vi "Colour sorting machine(all modules combined).vi"() -> ()   [LabVIEW 2018]
uses:
  <vilib>/userdefined/High Color/IMAQdx.ctl
  <vilib>/myRIO/Instrument Drivers/Onboard IO/DIO/typedefs/DIO Reference.ctl
  <vilib>/myRIO/Common/Instrument Driver Framework/Utilities/typedefs/myRIO Generic Hardware Reference.ctl
  <vilib>/myRIO/Common/Instrument Driver Framework/Utilities/typedefs/Hardware Version Enum.ctl
  <vilib>/myRIO/Common/Instrument Driver Framework/Utilities/typedefs/myRIO v1.0 Reference.ctl
  <vilib>/myRIO/Common/Instrument Driver Framework/Utilities/typedefs/Generic FPGA Reference.ctl
  <vilib>/myRIO/Common/Instrument Driver Framework/myRIO v1.0/DIO/typedefs/DIO Channels List.ctl
  <vilib>/myRIO/Common/Instrument Driver Framework/myRIO v1.0/DIO/typedefs/DIO Channels Enum.ctl
  <vilib>/userdefined/High Color/nirio_resource_hc.ctl
  <vilib>/myRIO/Instrument Drivers/Onboard IO/PWM/typedefs/PWM Reference.ctl
  <vilib>/myRIO/Common/Instrument Driver Framework/myRIO v1.0/PWM/typedefs/PWM Channels Enum.ctl
  <vilib>/myRIO/Instrument Drivers/Onboard IO/PWM/typedefs/PWM Configuration.ctl
  <vilib>/myRIO/Common/Instrument Driver Framework/Utilities/vis/Is FPGA Ref Available.vi
  <vilib>/myRIO/Common/Instrument Driver Framework/myRIO v1.0/DIO/vis/myRIO v1.1 Open DIO.vi
  <vilib>/myRIO/Instrument Drivers/Onboard IO/DIO/vis/Write.vi
  <vilib>/myRIO/Common/Instrument Driver Framework/myRIO v1.0/PWM/vis/myRIO v1.1 Open PWM.vi
  <vilib>/myRIO/Instrument Drivers/Onboard IO/PWM/vis/Set Duty Cycle and Frequency.vi
  <vilib>/myRIO/Common/Instrument Driver Framework/Utilities/vis/Validate Channels.vi
  <vilib>/myRIO/Common/Instrument Driver Framework/myRIO v1.0/DIO/vis/myRIO v1.0 Reserve DIO.vi
  <vilib>/myRIO/Common/Instrument Driver Framework/myRIO v1.0/PWM/vis/myRIO v1.0 Reserve PWM.vi
  <vilib>/myRIO/Common/Instrument Driver Framework/myRIO v1.0/Resource Manager/vis/myRIO v1.0 Reserve Channel List.vi
  <vilib>/myRIO/Common/Instrument Driver Framework/myRIO v1.0/DIO/vis/myRIO v1.0 Build MUX Configuration DIO.vi
  <vilib>/myRIO/Common/Instrument Driver Framework/myRIO v1.0/PWM/vis/myRIO v1.0 Build MUX Configuration PWM.vi
  <vilib>/myRIO/Common/Instrument Driver Framework/myRIO v1.0/Resource Manager/vis/myRIO v1.0 Reserve Channel.vi
  <vilib>/myRIO/Common/Instrument Driver Framework/myRIO v1.0/Resource Manager/vis/myRIO v1.0 Unreserve Channel.vi
  <vilib>/myRIO/Common/Instrument Driver Framework/myRIO v1.0/Resource Manager/vis/myRIO v1.0 Create Configuration List.vi
  <vilib>/myRIO/Common/Instrument Driver Framework/myRIO v1.0/Resource Manager/vis/myRIO v1.0 Build Mutex Name.vi
  <vilib>/Utility/VariantDataType/GetNumericInfo.vi
  <vilib>/Utility/error.llb/Error Cluster From Error Code.vi
  <vilib>/myRIO/Common/Instrument Driver Framework/myRIO v1.0/myRIO v1.1 Open.vi
  <vilib>/myRIO/Common/Instrument Driver Framework/Utilities/vis/IO Manager.vi
  <vilib>/myRIO/Common/Instrument Driver Framework/Utilities/vis/Configuration Manager.vi
  <vilib>/myRIO/Common/Instrument Driver Framework/myRIO v1.0/Resource Manager/vis/myRIO v1.0 Configure IO.vi
  <vilib>/myRIO/Common/Instrument Driver Framework/myRIO v1.0/myRIO v1.0 Close.vi
  <vilib>/myRIO/Common/Instrument Driver Framework/myRIO v1.0/DIO/vis/myRIO v1.0 Write DIO.vi
  <vilib>/myRIO/Common/Instrument Driver Framework/myRIO v1.0/PWM/vis/myRIO v1.0 Write PWM.vi
  <vilib>/myRIO/Express VI/Onboard IO/DO/DO Express VI.xnode
  <vilib>/myRIO/Instrument Drivers/Onboard IO/DIO/vis/myRIO DIO Open.xnode
  <vilib>/myRIO/Express VI/Onboard IO/PWM/PWM Express VI.xnode
  <vilib>/myRIO/Instrument Drivers/Onboard IO/PWM/vis/myRIO PWM Open.xnode
  <vilib>/myRIO/Instrument Drivers/Onboard IO/DIO/DIO.lvlib
  <vilib>/myRIO/Instrument Drivers/Onboard IO/PWM/PWM.lvlib
  <vilib>/vision/driver/NI_Vision_Acquisition_Software.lvlib
  <vilib>/vision/NI_Vision_Development_Module.lvlib
panel:
  out "Image":T1(plugin-control)
  out "red":bool
  out "blue":bool
  out "green":bool
  in  "Color Sensitivity":u32(ring) items=["Low", "Medium", "High"]
  out "Color Spectrum":dbl[](array[numeric]) format="%.2f"
  in  "Frequency [Hz]":dbl=1000.0
  in  "Duty Cycle":dbl=0.5297619047619048
  out "Numeric 3":i32
  out "x = y?":bool
  out "Numeric 2":i32
  out "Boolean":bool
  in  "stop":bool
  # "green"
  # "red"
  # "blue"
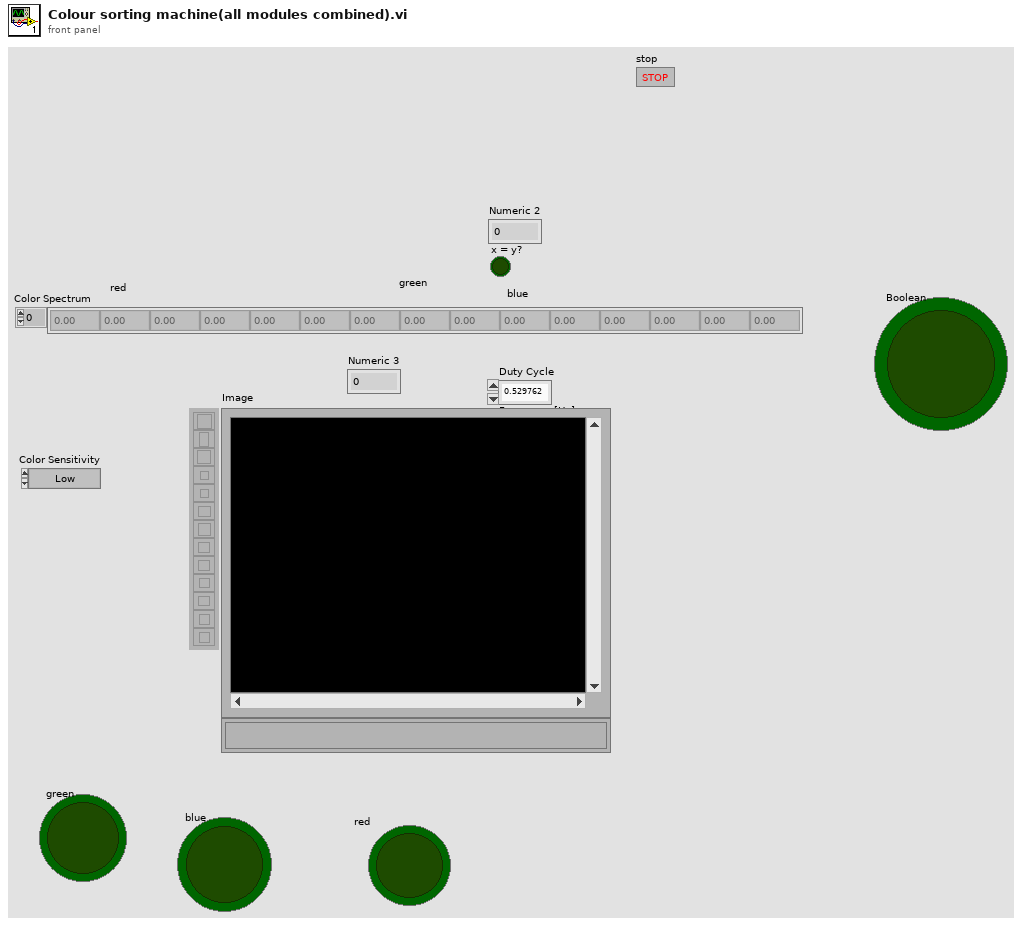
[diagram p1: front panel]
types:
  T1 = typedef "IMAQ Image.ctl" = refnum<image>
  T2 = typedef "IMAQdx.ctl" = refnum<k21>
  T3 = typedef "DIO.lvlib/DIO Reference.ctl" = cluster{"myRIO Reference":T4, "DIO Channels List":T8}
  T4 = typedef "myRIO Generic Hardware Reference.ctl" = cluster{"myRIO Model":T5, "myRIO Hardware Reference":T6}
  T5 = typedef "Hardware Version Enum.ctl" = enum16{"Unknown", "myRIO-1900", "myRIO-1950", "roboRIO", "NI ELVIS RIO CM", "ELVIS III"}
  T6 = typedef "myRIO v1.0 Reference.ctl" = cluster{"Generic FPGA Reference":T7, "Allow multiple opens":bool}
  T7 = typedef "Generic FPGA Reference.ctl" = refnum<k20>
  T8 = typedef "DIO Channels List.ctl" = T9[]
  T9 = typedef "DIO Channels Enum.ctl" = enum16{"Not Connected", "C/DIO0", "C/DIO1", "C/DIO2", "C/DIO3", "C/DIO4", "C/DIO5", "C/DIO6", "C/DIO7", "A/DIO0", "A/DIO1", "A/DIO2", "A/DIO3", "A/DIO4", "A/DIO5", "A/DIO6", "A/DIO7", "A/DIO8", "A/DIO9", "A/DIO10", "A/DIO11", "A/DIO12", "A/DIO13", "A/DIO14", "A/DIO15", "A/DIO16", "A/DIO17", "A/DIO18", "A/DIO19", "B/DIO0", "B/DIO1", "B/DIO2", "B/DIO3", "B/DIO4", "B/DIO5", "B/DIO6", "B/DIO7", "B/DIO8", "B/DIO9", "B/DIO10", "B/DIO11", "B/DIO12", "B/DIO13", "B/DIO14", "B/DIO15", "B/DIO16", "B/DIO17", "B/DIO18", "B/DIO19", "LED0", "LED1", "LED2", "LED3", "Button0", "DIO/DIO0", "DIO/DIO1", "DIO/DIO2", "DIO/DIO3", "DIO/DIO4", "DIO/DIO5", "DIO/DIO6", "DIO/DIO7", "DIO/DIO8", "DIO/DIO9", "SPI/CS0", "SPI/CS1", "SPI/CS2", "SPI/CS3", "LED RADIO (Green)", "LED RADIO (Red)", "LED COMM (Green)", "LED COMM (Red)", "LED MODE (Green)", "LED MODE (Red)"}
  T10 = typedef "nirio_resource_hc.ctl" = tag
  T11 = typedef "PWM.lvlib/PWM Reference.ctl" = cluster{"myRIO Reference":T4, "PWM Channels Enum":T12, "PWM Configuration":T13}
  T12 = typedef "PWM Channels Enum.ctl" = enum16{"Not Connected", "C/PWM0", "C/PWM1", "A/PWM0", "A/PWM1", "A/PWM2", "A/PWM3", "A/PWM4", "A/PWM5", "A/PWM6", "A/PWM7", "A/PWM8", "A/PWM9", "A/PWM10", "A/PWM11", "A/PWM12", "A/PWM13", "A/PWM14", "A/PWM15", "A/PWM16", "A/PWM17", "A/PWM18", "A/PWM19", "B/PWM0", "B/PWM1", "B/PWM2", "B/PWM3", "B/PWM4", "B/PWM5", "B/PWM6", "B/PWM7", "B/PWM8", "B/PWM9", "B/PWM10", "B/PWM11", "B/PWM12", "B/PWM13", "B/PWM14", "B/PWM15", "B/PWM16", "B/PWM17", "B/PWM18", "B/PWM19", "PWM/PWM0", "PWM/PWM1", "PWM/PWM2", "PWM/PWM3", "PWM/PWM4", "PWM/PWM5", "PWM/PWM6", "PWM/PWM7", "PWM/PWM8", "PWM/PWM9"}
  T13 = typedef "PWM.lvlib/PWM Configuration.ctl" = cluster{"Frequency":dbl, "Duty Cycle":dbl}
  T14 = cluster{"Global Rectangle":i32[], "Contours":cluster{"Contour Type":u32, "ROI Type":u32, "Points":i32[]}[]}
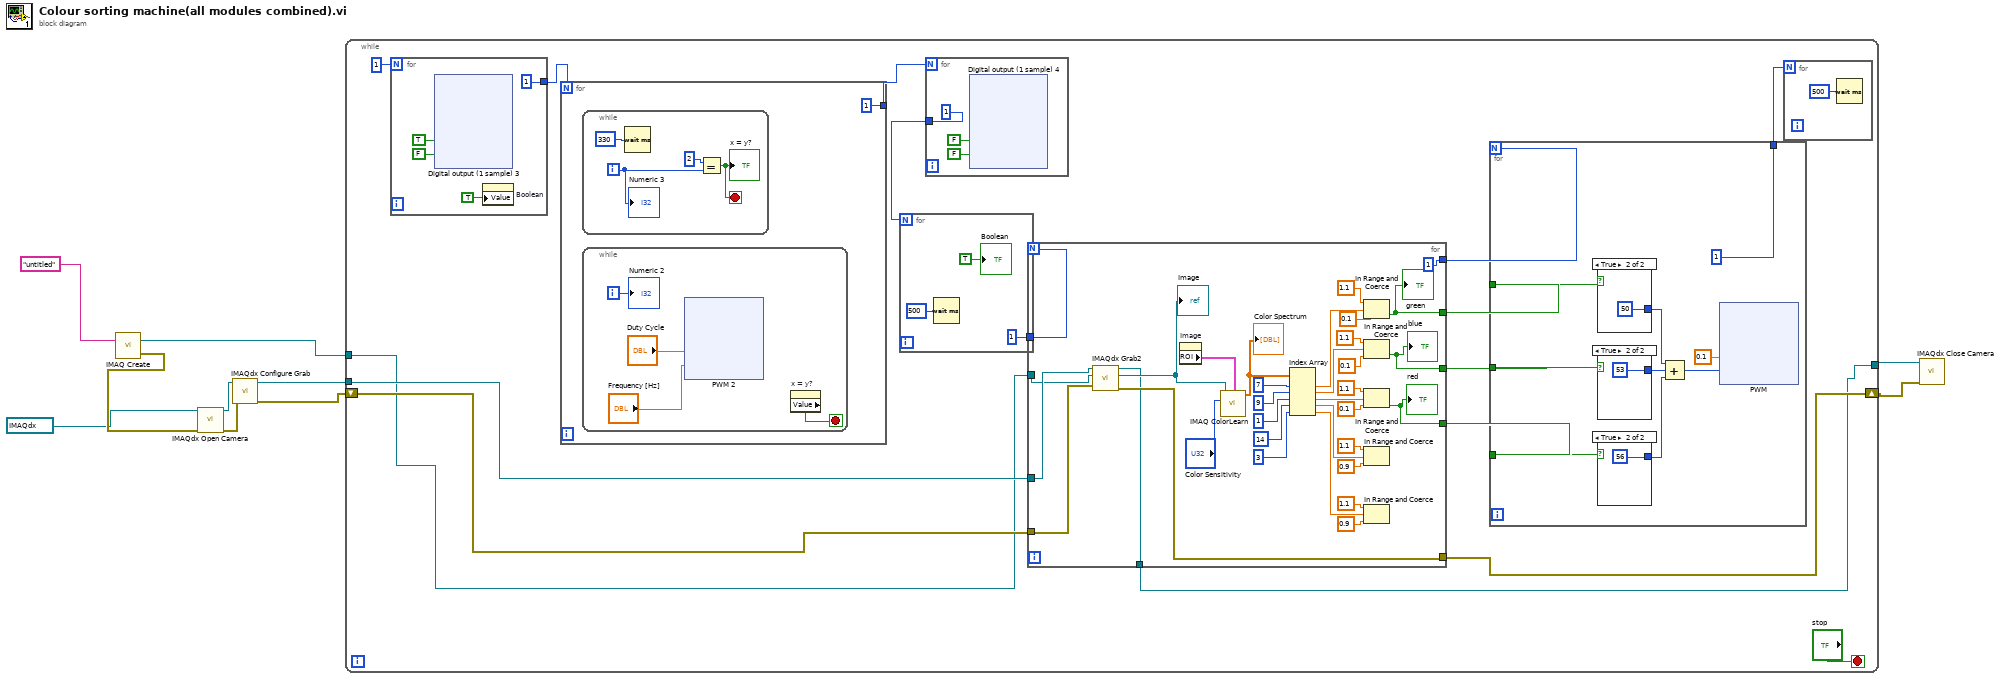
[diagram p0: block diagram]
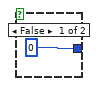
[diagram p4: hidden frame]
diagram:
  n1 = call "IMAQ Create"("Image Name"="untitled") -> ("New Image"=w3:T1, "error out"=w10:errorcluster)  [unwired: 4 in]
  n2 = call <vilib>:"IMAQdx Open Camera.vi"("error in"=w10, "Session In"=T2 "cam0") -> ("error out"=w8:errorcluster, "Session Out"=w9:T2)  [unwired: 8 in]
  n3 = call <vilib>:"IMAQdx Configure Grab.vi"("error in"=w8, "Session In"=w9) -> ("error out"=w5:errorcluster, "Session Out"=w4:T2)  [unwired: 8 in]
  n4 = while {
    shift-right: [w17] -> w2
    shift-left: w5 -> [w20]
    tunnel: w4 -> [w19]
    tunnel: w3 -> [w18]
    tunnel: [w16] -> w1
    stop <- "stop" stop-if-true
    n5 = for {
      N: 1 -> [_]
      tunnel: [1] -> w23
      n6 = xnode "Digital output (1 sample) 3"("clock (B/DIO0 (Pin 11))"=TRUE, "AntiClock (B/DIO1 (Pin 13))"=FALSE) -> ()  [unwired: 1 in, 1 out]
      n7 = property on="Boolean" class="Bool (strict)"("Value"=TRUE) -> ()  [unwired: 2 in, 2 out]
    }
    n8 = for {
      N: w23 -> [_]
      tunnel: [1] -> w22
      n9 = while {
        i -> [w70]
        stop <- w68 stop-if-true
        n10 = Wait (ms)(milliseconds to wait=u32 330) -> ()  [unwired: 1 out]
        n11 = Equal?(x=2, y=w70) -> (x = y?=w68:bool)
        "x = y?" <- w68
        "Numeric 3" <- w70
      }
      n12 = while {
        i -> [w75]
        stop <- w74 stop-if-true
        n13 = xnode "PWM 2"("Duty Cycle"="Duty Cycle", "Frequency [Hz]"="Frequency [Hz]") -> ()  [unwired: 1 in, 1 out]
        n14 = property on="x = y?" class="Bool (strict)"() -> ("Value"=w74:bool)  [unwired: 2 in, 2 out]
        "Numeric 2" <- w75
      }
    }
    n15 = for {
      N: w22 -> [_]
      tunnel: [1] -> w15
      n16 = xnode "Digital output (1 sample) 4"("clock (B/DIO0 (Pin 11))"=FALSE, "AntiClock (B/DIO1 (Pin 13))"=FALSE) -> ()  [unwired: 1 in, 1 out]
    }
    n17 = for {
      N: w15 -> [_]
      tunnel: [1] -> w25
      n18 = Wait (ms)(milliseconds to wait=u32 500) -> ()  [unwired: 1 out]
      "Boolean" <- TRUE
    }
    n19 = for {
      N: w25 -> [_]
      tunnel: [1] -> w21
      tunnel: w20 -> [w211]
      tunnel: w19 -> [w210]
      tunnel: w18 -> [w209]
      tunnel: [w208] -> w17
      tunnel: [w207] -> w16
      tunnel: [w206] -> w14
      tunnel: [w205] -> w13
      tunnel: [w204] -> w12
      n20 = call <vilib>:"IMAQdx Grab2.vi"("error in"=w211, "Image In"=w209, "Session In"=w210) -> ("error out"=w208:errorcluster, "Image Out"=w214:T1, "Session Out"=w207:T2)  [unwired: 5 in, 1 out]
      "Image" <- w214
      n21 = property on="Image" class="ImageControl"() -> ("ROI"=w213:T14)  [unwired: 2 in, 2 out]
      n22 = call "IMAQ ColorLearn"("ROI Descriptor"=w213, "Image"=w214, "Color Sensitivity"="Color Sensitivity") -> ("Color Spectrum"=w233:dbl[])  [unwired: 5 in, 1 out]
      "Color Spectrum" <- w233
      n23 = Index Array(array=w233, index #1=7 ("index"), index #2=9 ("index"), index #3=1 ("index"), index #4=14 ("index"), index #5=3 ("index")) -> (element #1=w203:dbl, element #2=w226:dbl, element #3=w223:dbl, element #4=w220:dbl, element #5=w218:dbl)
      n24 = In Range and Coerce(upper limit=1.1, x=w203, lower limit=0.1) -> (In Range?=w206:bool)  [unwired: 1 out]
      "green" <- w206
      n25 = In Range and Coerce(upper limit=1.1, x=w226, lower limit=0.1) -> (In Range?=w205:bool)  [unwired: 1 out]
      "blue" <- w205
      n26 = In Range and Coerce(upper limit=1.1, x=w223, lower limit=0.1 ("element")) -> (In Range?=w204:bool)  [unwired: 1 out]
      "red" <- w204
      n27 = In Range and Coerce(upper limit=1.1, x=w220, lower limit=0.9) -> ()  [unwired: 2 out]
      n28 = In Range and Coerce(upper limit=1.1, x=w218, lower limit=0.9) -> ()  [unwired: 2 out]
    }
    n29 = for {
      N: w21 -> [_]
      tunnel: w14 -> [w157]
      tunnel: w13 -> [w156]
      tunnel: w12 -> [w155]
      tunnel: [1] -> w11
      n30 = case shown="True" w157 {
        tunnel: [0 50] -> w162
        frame False {
        }
        frame True {
        }
      }
      n31 = case shown="True" w156 {
        tunnel: [_ 53] -> w161
        frame False {
        }
        frame True {
        }
      }
      n32 = case shown="True" w155 {
        tunnel: [_ 56] -> w160
        frame False {
        }
        frame True {
        }
      }
      n33 = Compound Arithmetic op=ADD(w162, w161, w160) -> (w154:i32)
      n34 = xnode "PWM"("Duty Cycle"=0.1 ("Knob"), "Frequency [Hz]"=w154) -> ()  [unwired: 1 in, 1 out]
    }
    n35 = for {
      N: w11 -> [_]
      n36 = Wait (ms)(milliseconds to wait=u32 500) -> ()  [unwired: 1 out]
    }
  }
  n37 = call <vilib>:"IMAQdx Close Camera.vi"("error in"=w2, "Session In"=w1) -> ()  [unwired: 9 in, 1 out]
